vi "decodeDataIdentity.vi"(5 "dataIdentityCode":string) -> (0 "unit":string, 1 "dataFormat":string, 2 "dataIdentityText":string)   [LabVIEW 2010]
uses:
  <vilib>/xml/Load XML File.vi
  <vilib>/xml/NI_XML.lvlib
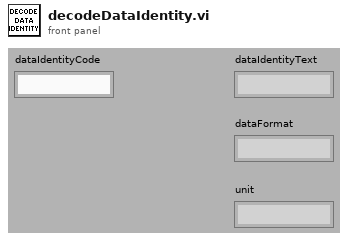
[diagram p1: front panel]
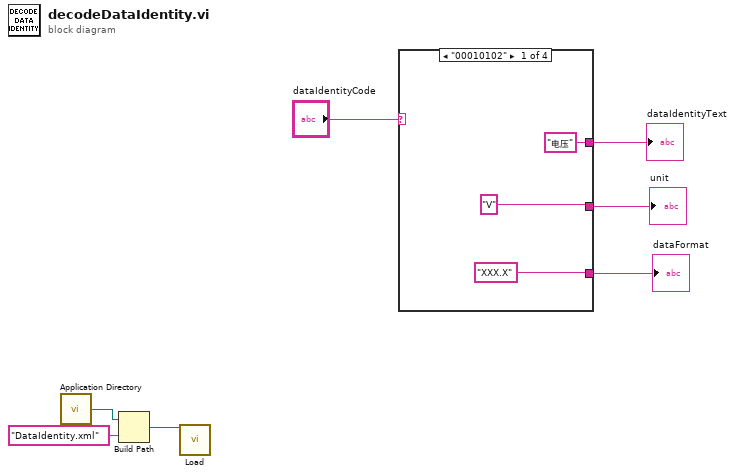
[diagram p0: block diagram]
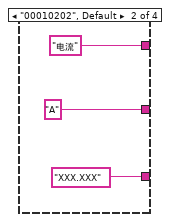
[diagram p2: hidden frame]
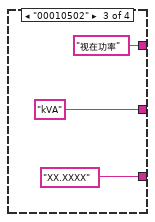
[diagram p3: hidden frame]
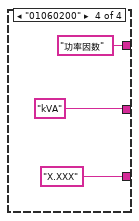
[diagram p4: hidden frame]
diagram:
  n1 = call <vilib>:"Application Directory.vi"() -> ("Application Directory"=w5:path)
  n2 = Build Path(base path=w5, name or relative path="DataIdentity.xml") -> (appended path=w3:path)
  n3 = call-poly <vilib>:"Load.vi"("path to XML document"=w3) -> ()  [unwired: 12 in, 3 out]
  n4 = case shown="\"00010102\"" "dataIdentityCode" {
    tunnel: ["电压" "电流" "视在功率" "功率因数"] -> w6
    tunnel: ["V" "A" "kVA" "kVA"] -> w2
    tunnel: ["XXX.X" "XXX.XXX" "XX.XXXX" "X.XXX"] -> w1
    frame "00010102" {
    }
    frame "00010202", Default {
    }
    frame "00010502" {
    }
    frame "01060200" {
    }
  }
  "dataIdentityText" <- w6
  "unit" <- w2
  "dataFormat" <- w1
